vi "ID Parser.vi"(8 "error in (no error)":errorcluster, 10 "ID":string, 11 "Lutron QS Object in":refnum<class "Lutron QS Object.lvclass">) -> (0 "error out":errorcluster, 3 "Lutron QS Object out":refnum<class "Lutron QS Object.lvclass">)   [LabVIEW 2016, in "Lutron QS Control Protocol.lvlib" / "Lutron QS Object.lvclass"]
uses:
  Lutron QS Object.lvclass
panel:
  out "Array - String 2":string[](array[string])
  out "Array - String":string[](array[string])
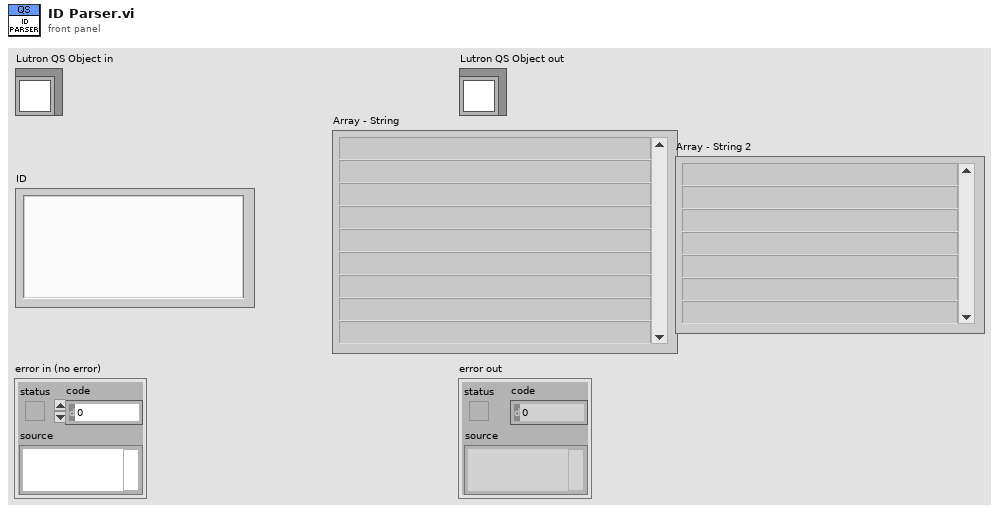
[diagram p1: front panel]
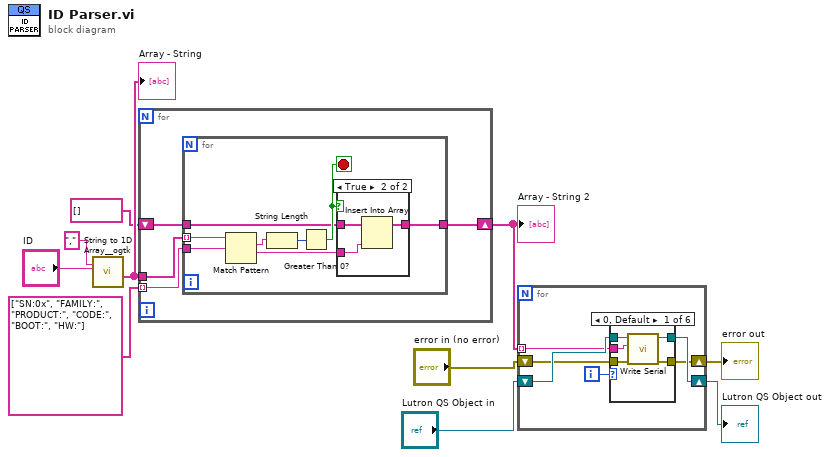
[diagram p0: block diagram]
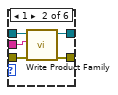
[diagram p2: hidden frame]
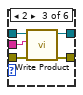
[diagram p3: hidden frame]
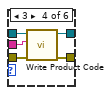
[diagram p4: hidden frame]
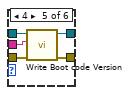
[diagram p5: hidden frame]
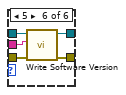
[diagram p6: hidden frame]
diagram:
  n1 = call <userlib>:"String to 1D Array__ogtk.vi"("delimiter (Tab)"=",", "string"="ID") -> ("Array of Strings"=w7:string[])  [unwired: 9 in]
  "Array - String" <- w7
  n2 = for {
    tunnel: string[] ["SN:0x", "FAMILY:", "PRODUCT:", "CODE:", "BOOT:", "HW:"] -> [w13] mode=indexing
    tunnel: w7 -> [w14]
    shift-right: [w11] -> w5
    shift-left: string[] [] -> [w12]
    n3 = for {
      tunnel: w14 -> [w22] mode=indexing
      tunnel: w13 -> [w21]
      tunnel: w12 -> [w18]
      tunnel: [w16] -> w11
      stop <- w19 stop-if-true
      n4 = Match Pattern(string=w22, regular expression=w21) -> (match substring=w17:string, after substring=w15:string)  [unwired: 1 in, 2 out]
      n5 = String Length(string=w17) -> (length=w20:i32)
      n6 = Greater Than 0?(x=w20) -> (x > 0?=w19:bool)
      n7 = case shown="True" w19 {
        tunnel: w18 -> [w23 w26]
        tunnel: w15 -> [_ w25]
        tunnel: [w23 w24] -> w16
        frame False {
        }
        frame True {
          n8 = Insert Into Array(array=w26, new element=w25) -> (w24:string[])  [unwired: 1 in]
        }
      }
    }
  }
  "Array - String 2" <- w5
  n9 = for {
    tunnel: w5 -> [w27] mode=indexing
    shift-right: [w30] -> w2
    shift-left: "Lutron QS Object in" -> [w31]
    shift-right: [w29] -> w1
    shift-left: "error in (no error)" -> [w28]
    i -> [w32]
    n10 = case shown="0, Default" w32 {
      tunnel: w31 -> [w37 w42 w47 w51 w57 w62]
      tunnel: [w35 w41 w43 w49 w54 w59] -> w30
      tunnel: [w33 w40 w44 w48 w53 w58] -> w29
      tunnel: w28 -> [w34 w39 w45 w50 w56 w61]
      tunnel: w27 -> [w36 w38 w46 w52 w55 w60]
      frame 0, Default {
        n11 = call-dynamic "Write Serial.vi"("error in (no error)"=w34, "Serial"=w36, "Generic Device in"=w37) -> ("error out"=w33:errorcluster, "Generic Device out"=w35:refnum<class "Lutron QS Object.lvclass">)  [unwired: 7 in]
      }
      frame 1 {
        n12 = call-dynamic "Write Product Family.vi"("error in (no error)"=w39, "Product Family"=w38, "Lutron QS Object in"=w42) -> ("error out"=w40:errorcluster, "Lutron QS Object out"=w41:refnum<class "Lutron QS Object.lvclass">)  [unwired: 7 in]
      }
      frame 2 {
        n13 = call-dynamic "Write Product.vi"("error in (no error)"=w45, "Product"=w46, "Lutron QS Object in"=w47) -> ("error out"=w44:errorcluster, "Lutron QS Object out"=w43:refnum<class "Lutron QS Object.lvclass">)  [unwired: 7 in]
      }
      frame 3 {
        n14 = call-dynamic "Write Product Code.vi"("error in (no error)"=w50, "Product Code"=w52, "Lutron QS Object in"=w51) -> ("error out"=w48:errorcluster, "Lutron QS Object out"=w49:refnum<class "Lutron QS Object.lvclass">)  [unwired: 7 in]
      }
      frame 4 {
        n15 = call-dynamic "Write Boot code Version.vi"("error in (no error)"=w56, "Boot code Version"=w55, "Lutron QS Object in"=w57) -> ("error out"=w53:errorcluster, "Lutron QS Object out"=w54:refnum<class "Lutron QS Object.lvclass">)  [unwired: 7 in]
      }
      frame 5 {
        n16 = call-dynamic "Write Software Version.vi"("error in (no error)"=w61, "Software Version"=w60, "Lutron QS Object in"=w62) -> ("error out"=w58:errorcluster, "Lutron QS Object out"=w59:refnum<class "Lutron QS Object.lvclass">)  [unwired: 7 in]
      }
    }
  }
  "error out" <- w1
  "Lutron QS Object out" <- w2
